vi "Main Loop.vi"(8 "error in (no error)":errorcluster, 11 "Sensor910 in":refnum<class "Sensor910.lvclass">) -> (0 "error out":errorcluster, 3 "Sensor910 out":refnum<class "Sensor910.lvclass">)   [LabVIEW 2020, in "Sensor910.lvclass"]
uses:
  Sensor910.lvclass
  <vilib>/Platform/TimedLoop/XDataNode/timing_clust.ctl
  <vilib>/Platform/TimedLoop/XDataNode/nitl_modes.ctl
  <vilib>/Platform/TimedLoop/XDataNode/wakeup.ctl
  Mode.ctl
  Command.ctl
  Settings.ctl
  Data.ctl
  9cfac15d-a9dc-4770-b8f0-68bacdc79c0f.vi
  94e3c92e-fcfa-43cb-ae47-d3a486abf537.vi
  b96c5f6a-59cc-4a84-9d2d-c86ca5fc82ce.vi
  9a13b59e-eb46-41c8-aff0-b09d3ab633f4.vi
  <vilib>/Platform/TimedLoop/scheduler/LVUserAPI/_suppVIs/Create_1kHz_TSource.vi
  <vilib>/NI Modbus.llb/MB Serial Master Query Write Single Register (poly).vi
  <vilib>/NI Modbus.llb/MB Serial Master Query Read Holding Registers (poly).vi
  <vilib>/NI Modbus.llb/MB Serial Master Query Read Input Registers (poly).vi
  <vilib>/platform/TimedLoop/XDataNode/XDataNode.xnode
  <vilib>/ErrorRing/Error Ring.xnode
  <vilib>/Platform/TimedLoop/XDataNode/XDNodeRunTimeDep.lvlib
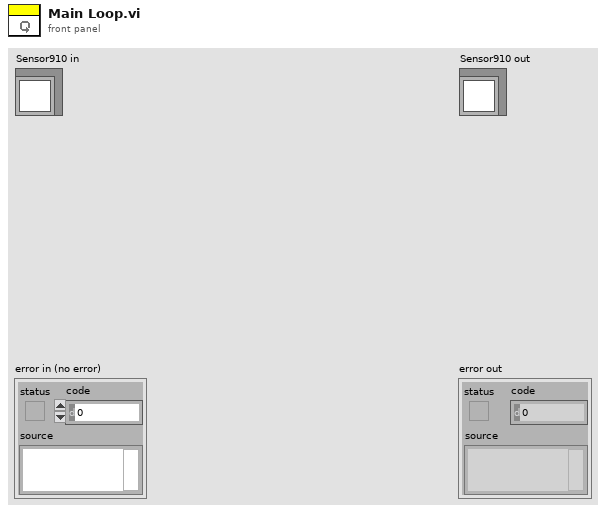
[diagram p1: front panel]
types:
  T1 = cluster{"Serial Parameters":cluster{"Mode":enum16{"RTU", "ASCII"}, "Slave Address":u8}, "VISA resource name":refnum<visa-resource-name>, "Period":i64, "Data Registers":u16[]}
  T2 = typedef "Sensor910.lvclass/Command.ctl" = cluster{"Address":u16, "Data":u16}
  T3 = typedef "Sensor910.lvclass/Settings.ctl" = cluster{"Serial Parameters":cluster{"Mode":enum16{"RTU", "ASCII"}, "Slave Address":u8}, "VISA resource name":refnum<visa-resource-name>, "Period":i64, "Data Registers":u16[], "Baud Rate":u32}
  T4 = typedef "Sensor910.lvclass/Data.ctl" = cluster{"Connect":bool, "No Response":bool, "Data":sgl[]}
  T5 = cluster{"Mode":enum16{"RTU", "ASCII"}, "Slave Address":u8}
  T6 = typedef "Sensor910.lvclass/Mode.ctl" = enum16{"Inactiv", "Read Data", "Service Mode", "Enter offset", "Open session", "Close session", "Set Modbus Address", "Abort"}
  T7 = typedef "XDNodeRunTimeDep.lvlib/timing_clust.ctl" = cluster{"Expected End [f-1]":u64, "Actual End [f-1]":u64, "Finished Late? [f-1]":bool, "Expected End [i-1]":u64, "Actual End [i-1]":u64, "Finished Late? [i-1]":bool, "Expected Start [i]":u64, "Actual Start [i]":u64, "Expected Start [f]":u64, "Actual Start [f]":u64, "Source Name":string, "Structure Name":string, "Period":i64, "Deadline":i64, "Offset":i64, "Start":i64, "Priority":i32, "Timeout":i32, "Mode":T8, "Wakeup Reason":T9, "Error":errorcluster, "Source Type":string, "Secondary Source Type":string, "Global End Time":u64, "Global Start Time":u64, "Frame Duration":u64, "Iteration Duration":u64, "Assigned CPU":i32, "I/O Scan Engine Mode":u32}
  T8 = typedef "XDNodeRunTimeDep.lvlib/nitl_modes.ctl" = enum32{"No Change", "Process missed periods, maintain original phase", "Discard missed periods, maintain original phase", "Process missed periods, ignore original phase", "Discard missed periods, ignore original phase"}
  T9 = typedef "XDNodeRunTimeDep.lvlib/wakeup.ctl" = enum32{"Normal", "Aborted", "Asynchronous wakeup", "Timing source error", "Timed loop error", "Timeout"}
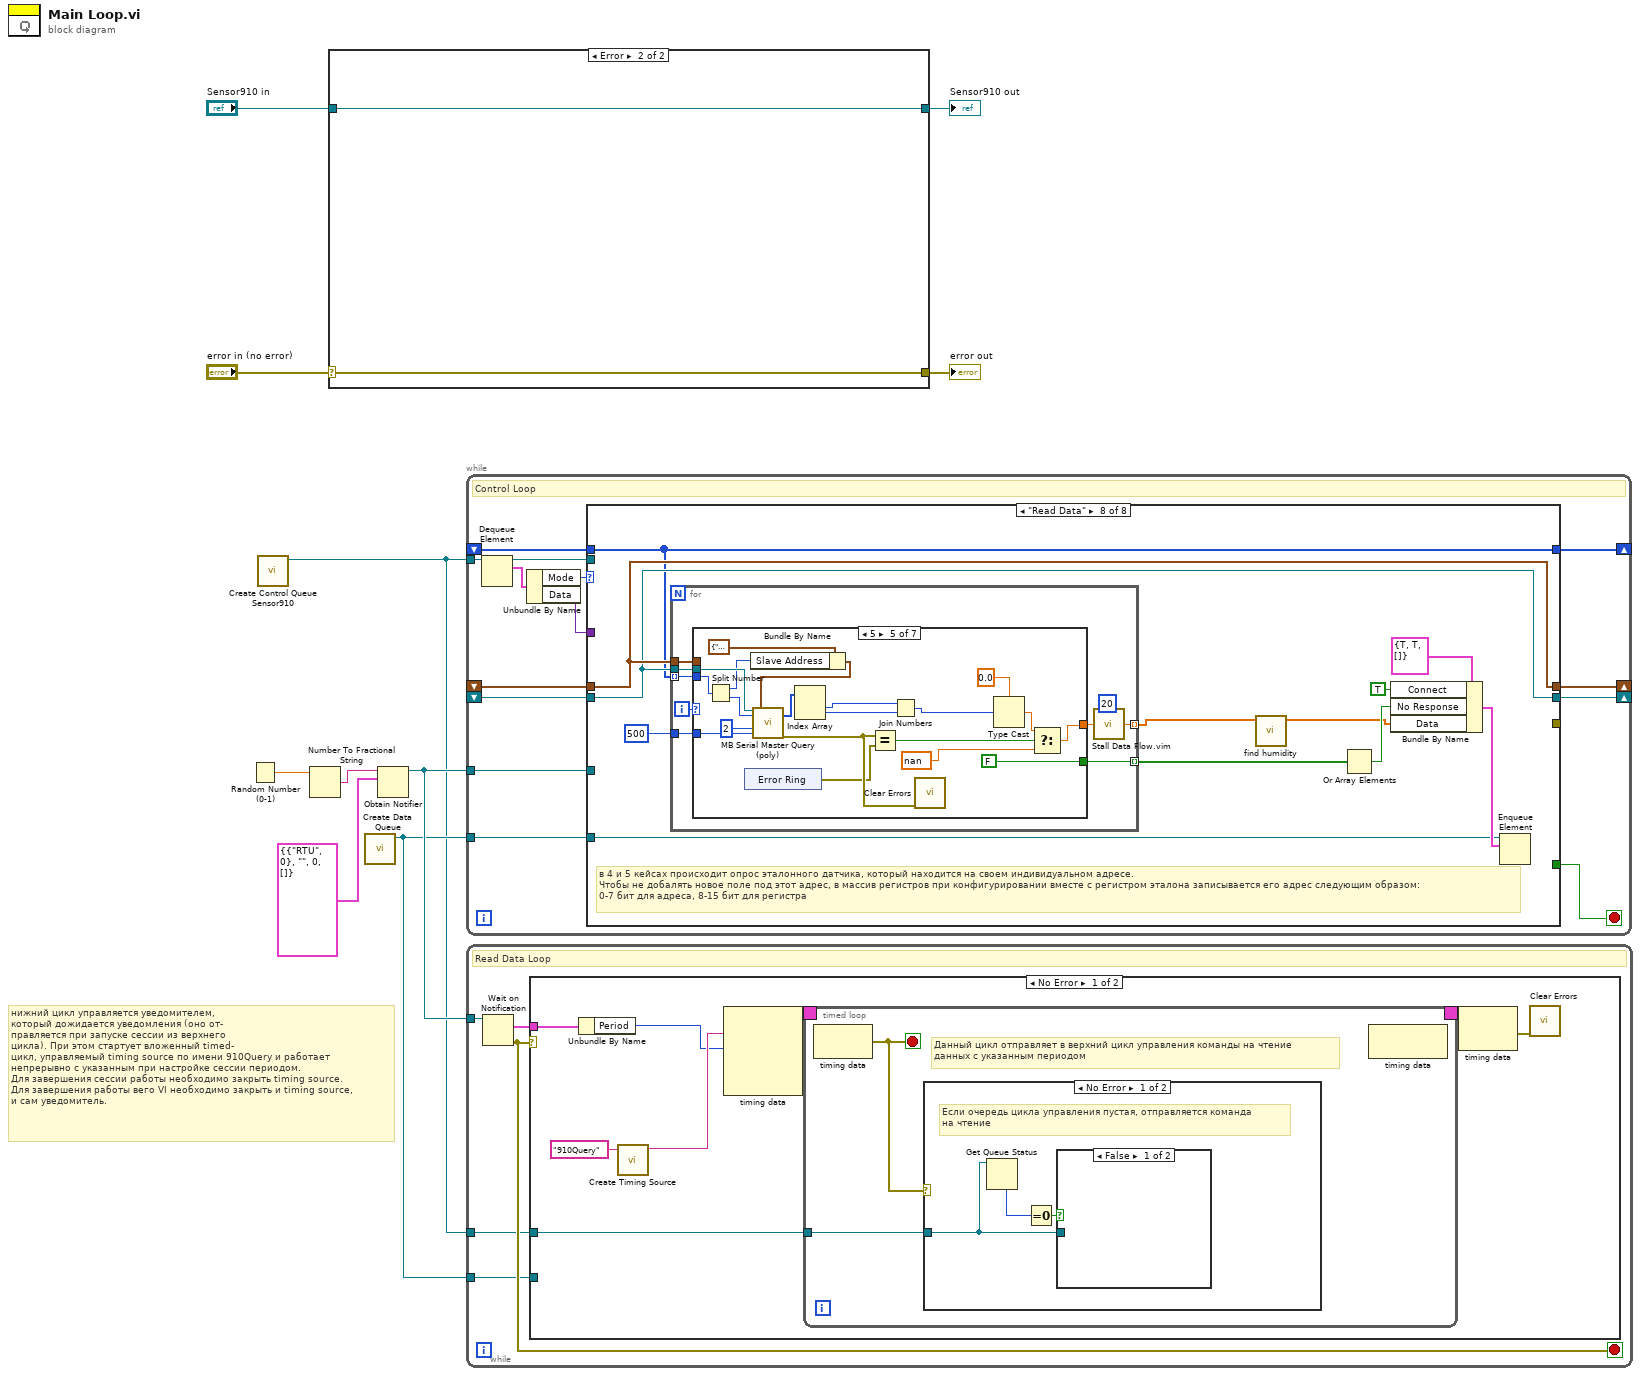
[diagram p0: block diagram]
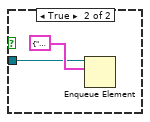
[diagram p2: hidden frame]
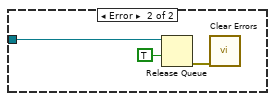
[diagram p4: hidden frame]
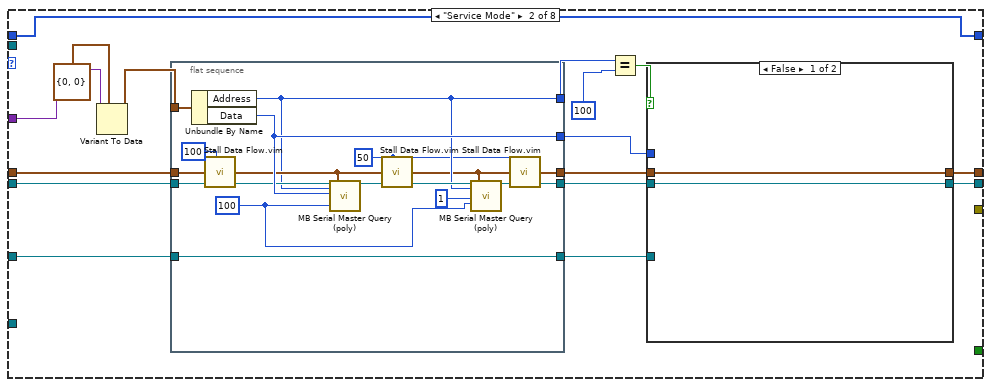
[diagram p6: hidden frame]
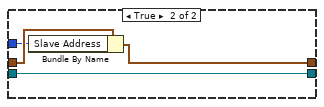
[diagram p7: hidden frame]
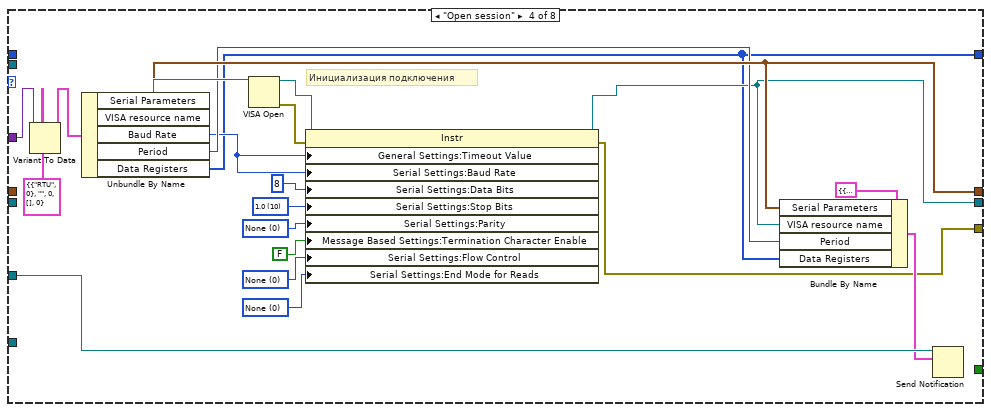
[diagram p9: hidden frame]
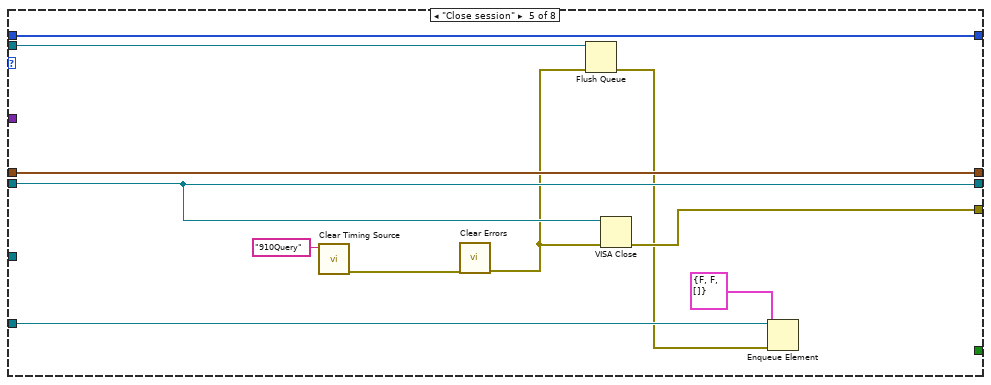
[diagram p10: hidden frame]
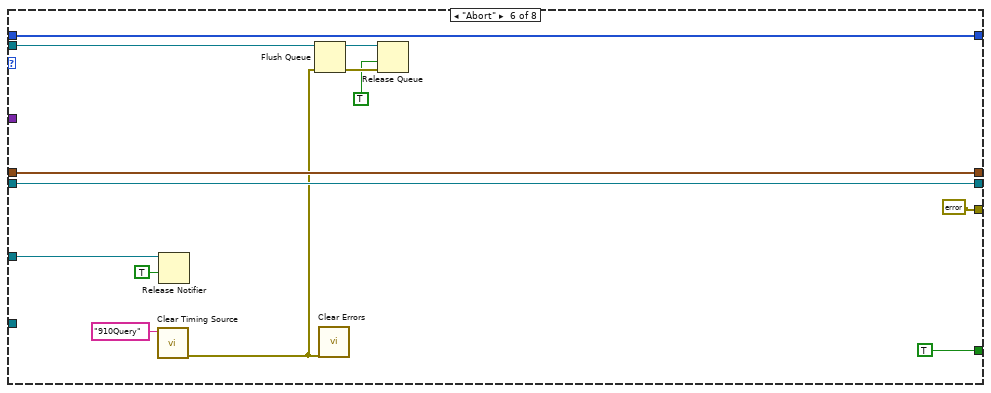
[diagram p11: hidden frame]
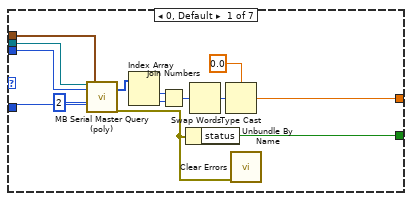
[diagram p13: hidden frame]
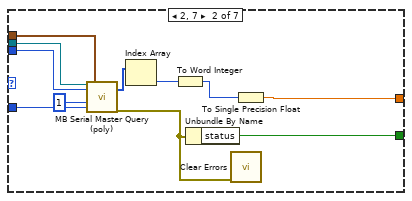
[diagram p14: hidden frame]
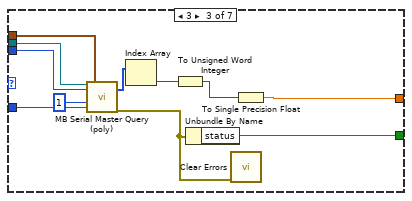
[diagram p15: hidden frame]
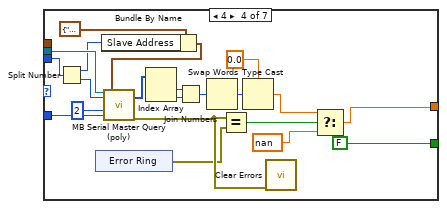
[diagram p16: hidden frame]
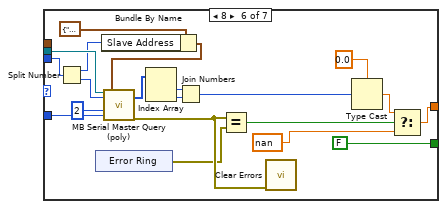
[diagram p17: hidden frame]
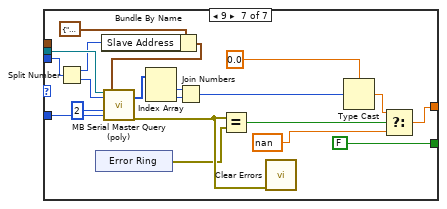
[diagram p18: hidden frame]
diagram:
  # "нижний цикл управляется уведомителем,\nкоторый дожидается уведомления (оно от-\nправляется при запуске сессии из верхнего\nцикла). При этом стартует вложенный timed-\nцикл, управляемый timing source по имени 910Query и работает\nнепрерывно с указанным при настройке сессии периодом.\nДля завершения сессии работы необходимо закрыть timing source.\nДля завершения работы вего VI необходимо закрыть и timing source,\nи сам уведомитель."
  n1 = Random Number (0-1)() -> (number: 0 to 1=w5:dbl)
  n2 = call "Create Control Queue Sensor910.vi"() -> ("queue out"=w1:refnum<queue>)  [unwired: 9 in, 2 out]
  n3 = Number To Fractional String(number=w5) -> (F-format string=w6:string)  [unwired: 3 in]
  n4 = case shown="Error" "error in (no error)" {
    selector: "error in (no error)" -> [w11 w14]
    tunnel: [w11 w14] -> w9
    tunnel: [w12 w13] -> w7
    tunnel: "Sensor910 in" -> [w12 w13]
    frame No Error {
      # "Wire the error cluster across even in the \"No Error\"\ncase so that warnings get propagated."
    }
    frame Error {
    }
  }
  "error out" <- w9
  "Sensor910 out" <- w7
  n5 = call "Create Data Queue.vi"() -> ("queue out"=w2:refnum<queue>)  [unwired: 10 in, 1 out]
  n6 = Obtain Notifier(name (unnamed)=w6, notification data type=T1 {"Serial Parameters"={"Mode"=enum."RTU", "Slave Address"=0}, "VISA resource name"="", "Period"=0, "Data Registers"=[]} ("Cluster")) -> (notifier out=w4:refnum<notifier>)  [unwired: 2 in, 2 out]
  n7 = while {
    tunnel: w1 -> [w28]
    tunnel: w4 -> [w25]
    shift-right: [w24] -> _
    shift-left: _ -> [w21]
    shift-right: [w23] -> _
    shift-left: _ -> [w20]
    shift-right: [w18] -> _
    shift-left: _ -> [w17]
    tunnel: w2 -> [w16]
    stop <- w19 stop-if-true
    # "Control Loop"
    n8 = Dequeue Element(queue=w28) -> (queue out=w15:refnum<queue>, element=w27:cluster{"Mode":T6, "Data":variant})  [unwired: 2 in, 2 out]
    n9 = Unbundle By Name(w27) -> ("Mode"=w26:T6, "Data"=w22:variant)
    n10 = case shown="\"Read Data\"" w26 {
      tunnel: w25 -> [_ w34 _ w83 _ w115 _ _]
      tunnel: [w31 w39 w71 w81 w101 w112 w118 w125] -> w24
      tunnel: [w30 w37 w70 w74 w100 w111 w119 w124] -> w23
      tunnel: w22 -> [_ w47 _ w79 _ _ _ _]
      tunnel: w21 -> [w31 w44 w71 _ w101 w112 w118 w125]
      tunnel: w20 -> [w30 w45 w70 _ w100 w111 w119 w124]
      tunnel: [_ _ _ w73 w99 errorcluster {"status"=TRUE, "code"=0, "source"=""} ("error out") _ _] -> _
      tunnel: [_ _ _ _ _ TRUE _ _] -> w19
      tunnel: [w29 w32 w69 w72 w98 w109 w117 w123] -> w18
      tunnel: w17 -> [w29 w32 w69 _ w98 w109 w117 w123]
      tunnel: w16 -> [_ _ _ _ w96 _ _ w122]
      tunnel: w15 -> [_ _ _ _ w95 w108 _ _]
      frame "Inactiv", Default {
      }
      frame "Service Mode" {
        n11 = Variant To Data(type=T2 {"Address"=0, "Data"=0} ("Command"), Variant=w47) -> (data=w43:T2)  [unwired: 1 in, 1 out]
        n12 = flat-sequence {
          tunnel: w45 -> [w63]
          tunnel: w44 -> [w65]
          tunnel: [w58] -> w36
          tunnel: w43 -> [w68]
          tunnel: [w56] -> w38
          tunnel: [w60] -> w42
          tunnel: [w67] -> w35
          tunnel: [w66] -> w33
          tunnel: w34 -> [w66]
          frame #0 {
            w55 = u32 50 ("milliseconds to wait")
            w54 = u32 100 ("Timeout")
            n13 = Unbundle By Name(w68) -> ("Address"=w60:u16, "Data"=w67:u16)
            n14 = call "Stall Data Flow.vim"("value in"=w65, "milliseconds to wait"=u32 100) -> ("value out"=w64:T5)  [unwired: 1 out]
            n15 = call-poly <vilib>:"MB Serial Master Query (poly).vi"("VISA resource name"=w63, "Address"=w60, "Holding Register"=w67, "Timeout"=w54, "Serial Parameters"=w64) -> ("VISA resource name out"=w61:refnum<visa-resource-name>)  [unwired: 12 in, 2 out]
            n16 = call "Stall Data Flow.vim"("value in"=w64, "milliseconds to wait"=w55) -> ("value out"=w57:T5)  [unwired: 1 out]
            n17 = call-poly <vilib>:"MB Serial Master Query (poly).vi"("VISA resource name"=w61, "Starting Address"=w60, "Quantity"=u16 1, "Timeout"=w54, "Serial Parameters"=w57) -> ("VISA resource name out"=w58:refnum<visa-resource-name>)  [unwired: 11 in, 3 out]
            n18 = call "Stall Data Flow.vim"("value in"=w57, "milliseconds to wait"=w55) -> ("value out"=w56:T5)  [unwired: 1 out]
          }
        }
        n19 = Equal?(x=w42, y=u16 100) -> (x = y?=w40:bool)
        n20 = case shown="False" w40 {
          tunnel: [w49 w50] -> w39
          tunnel: w38 -> [w49 w52]
          tunnel: [w48 w53] -> w37
          tunnel: w36 -> [w48 w53]
          tunnel: w35 -> [_ w51]
          tunnel: w33 -> [_ _]
          frame False {
          }
          frame True {
            n21 = Bundle By Name(cluster=w52, "Slave Address"=w51) -> (w50:T5)
          }
        }
      }
      frame "Enter offset" {
      }
      frame "Open session" {
        w92 = u16 0 items=["None", "Odd", "Even", "Mark", "Space"] ("Serial Settings:Parity")
        w91 = u16 0 items=["None", "XON/XOFF", "RTS/CTS", "XON/XOFF & RTS/CTS", "DTR/DSR", "XON/XOFF & DTR/DSR"] ("Serial Settings:Flow Control")
        w89 = u16 0 items=["None", "LastBit", "TermChar"] ("Serial Settings:Serial End Mode for Reads")
        w87 = u16 10 items=["1.0"=10, "1.5"=15, "2.0"=20] ("Serial Settings:Serial Stop Bits")
        # "Инициализация подключения"
        n22 = Variant To Data(type=T3 {"Serial Parameters"={"Mode"=enum."RTU", "Slave Address"=0}, "VISA resource name"="", "Period"=0, "Data Registers"=[], "Baud Rate"=0} ("Cluster"), Variant=w79) -> (data=w76:T3)  [unwired: 1 in, 1 out]
        n23 = Unbundle By Name(w76) -> ("Serial Parameters"=w81:T5, "VISA resource name"=w84:refnum<visa-resource-name>, "Baud Rate"=w77:u32, "Period"=w80:i64, "Data Registers"=w72:u16[])
        n24 = VISA Open(VISA resource name=w84) -> (VISA resource name=w86:refnum<visa-resource-name>, error out=w85:errorcluster)  [unwired: 4 in]
        n25 = property class="Instr"(reference=w86, error in=w85, "General Settings:Timeout Value"=w77, "Serial Settings:Baud Rate"=w77, "Serial Settings:Data Bits"=u16 8 ("data bits"), "Serial Settings:Stop Bits"=w87, "Serial Settings:Parity"=w92, "Message Based Settings:Termination Character Enable"=FALSE, "Serial Settings:Flow Control"=w91, "Serial Settings:End Mode for Reads"=w89) -> (reference out=w74:refnum<visa-resource-name>, error out=w73:errorcluster)
        n26 = Bundle By Name(cluster=T1 {"Serial Parameters"={"Mode"=enum."RTU", "Slave Address"=0}, "VISA resource name"="", "Period"=0, "Data Registers"=[]} ("notification"), "Serial Parameters"=w81, "VISA resource name"=w74, "Period"=w80, "Data Registers"=w72) -> (w75:T1)
        n27 = Send Notification(notification=w75, notifier=w83) -> ()  [unwired: 1 in, 2 out]
      }
      frame "Close session" {
        n28 = call <vilib>:"Clear Timing Source.vi"("name"="910Query" ("name (in)")) -> ("error out"=w102:errorcluster)  [unwired: 9 in, 1 out]
        n29 = call <vilib>:"Clear Errors.vi"("error in (no error)"=w102) -> ("error out"=w94:errorcluster)  [unwired: 5 in, 1 out]
        n30 = Flush Queue(queue=w95, error in (no error)=w94) -> (error out=w93:errorcluster)  [unwired: 2 out]
        n31 = VISA Close(VISA resource name=w100, error in (no error)=w94) -> (error out=w99:errorcluster)
        n32 = Enqueue Element(queue=w96, element=T4 {"Connect"=FALSE, "No Response"=FALSE, "Data"=[]}, error in (no error)=w93) -> ()  [unwired: 1 in, 3 out]
      }
      frame "Abort" {
        n33 = call <vilib>:"Clear Timing Source.vi"("name"="910Query" ("name (in)")) -> ("error out"=w107:errorcluster)  [unwired: 9 in, 1 out]
        n34 = Release Notifier(notifier=w115, force destroy? (F)=TRUE) -> ()  [unwired: 1 in, 3 out]
        n35 = Flush Queue(queue=w108, error in (no error)=w107) -> (queue out=w106:refnum<queue>, error out=w105:errorcluster)  [unwired: 1 out]
        n36 = call <vilib>:"Clear Errors.vi"("error in (no error)"=w107) -> ()  [unwired: 5 in, 2 out]
        n37 = Release Queue(queue=w106, force destroy? (F)=TRUE, error in (no error)=w105) -> ()  [unwired: 3 out]
      }
      frame "Set Modbus Address" {
      }
      frame "Read Data" {
        # "в 4 и 5 кейсах происходит опрос эталонного датчика, который находится на своем индивидуальном адресе.\nЧтобы не добалять новое поле под этот адрес, в массив регистров при конфигурировании вместе с регистром эталона записывается его адрес следующим образом:\n0-7 бит для адреса, 8-15 бит для регистра"
        n38 = for {
          tunnel: w125 -> [w140]
          tunnel: w124 -> [w139]
          tunnel: w123 -> [w138] mode=indexing
          tunnel: [w134] -> w130 mode=indexing
          tunnel: [w137] -> w128 mode=indexing
          tunnel: u32 500 ("Timeout") -> [w132]
          i -> [w136]
          n39 = case shown="5" w136 {
            tunnel: w140 -> [w154 w165 w176 _ _ _ _]
            tunnel: w139 -> [w153 w164 w175 w197 w218 w239 w260]
            tunnel: w138 -> [w152 w163 w174 w194 w215 w236 w257]
            tunnel: [w145 w158 w170 w179 w206 w224 w245] -> w135
            tunnel: [w143 w161 w173 FALSE ("status") FALSE ("status") FALSE ("status") FALSE ("status")] -> w137
            tunnel: w132 -> [w141 w155 w166 w177 w204 w222 w243]
            frame 0, Default {
              n40 = call-poly <vilib>:"MB Serial Master Query (poly).vi"("VISA resource name"=w153, "Starting Address"=w152, "Quantity"=u16 2, "Timeout"=w141, "Serial Parameters"=w154) -> ("Holding Registers"=w146:u16[], "error out"=w144:errorcluster)  [unwired: 11 in, 2 out]
              n41 = Index Array(array=w146) -> (element #1=w149:u16, element #2=w147:u16)  [unwired: 2 in]
              n42 = Join Numbers(hi=w149, lo=w147) -> ((hi.lo)=w151:u32)
              n43 = Unbundle By Name(w144) -> ("status"=w143:bool)
              n44 = Swap Words(1:w151) -> (0:w150:u32)
              n45 = Type Cast(type=sgl 0.0 ("p_atm"), x=w150) -> (*(type *) &x=w145:sgl)
              n46 = call <vilib>:"Clear Errors.vi"("error in (no error)"=w144) -> ()  [unwired: 5 in, 2 out]
            }
            frame 2, 7 {
              n47 = call-poly <vilib>:"MB Serial Master Query (poly).vi"("VISA resource name"=w164, "Starting Address"=w163, "Quantity"=u16 1, "Timeout"=w155, "Serial Parameters"=w165) -> ("Holding Registers"=w159:u16[], "error out"=w162:errorcluster)  [unwired: 11 in, 2 out]
              n48 = Index Array(array=w159) -> (element=w157:u16)  [unwired: 1 in]
              n49 = To Word Integer(number=w157) -> (16bit integer=w156:i16)
              n50 = Unbundle By Name(w162) -> ("status"=w161:bool)
              n51 = call <vilib>:"Clear Errors.vi"("error in (no error)"=w162) -> ()  [unwired: 5 in, 2 out]
              n52 = To Single Precision Float(number=w156) -> (single precision float=w158:sgl)
            }
            frame 3 {
              n53 = call-poly <vilib>:"MB Serial Master Query (poly).vi"("VISA resource name"=w175, "Starting Address"=w174, "Quantity"=u16 1, "Timeout"=w166, "Serial Parameters"=w176) -> ("Holding Registers"=w171:u16[], "error out"=w167:errorcluster)  [unwired: 11 in, 2 out]
              n54 = Index Array(array=w171) -> (element=w169:u16)  [unwired: 1 in]
              n55 = To Unsigned Word Integer(number=w169) -> (unsigned 16bit integer=w168:u16)
              n56 = Unbundle By Name(w167) -> ("status"=w173:bool)
              n57 = call <vilib>:"Clear Errors.vi"("error in (no error)"=w167) -> ()  [unwired: 5 in, 2 out]
              n58 = To Single Precision Float(number=w168) -> (single precision float=w170:sgl)
            }
            frame 4 {
              n59 = Split Number(x=w194) -> (hi(x)=w193:u8, lo(x)=w192:u8)
              n60 = xnode "Error Ring"() -> ("error out"=w182:errorcluster)
              n61 = Bundle By Name(cluster=T5 {"Mode"=enum."RTU", "Slave Address"=0} ("Serial Parameters"), "Slave Address"=w193) -> (w191:T5)
              n62 = call-poly <vilib>:"MB Serial Master Query (poly).vi"("VISA resource name"=w197, "Starting Address"=w192, "Quantity"=u16 2, "Timeout"=w177, "Serial Parameters"=w191) -> ("Input Registers"=w185:u16[], "error out"=w183:errorcluster)  [unwired: 11 in, 2 out]
              n63 = Index Array(array=w185) -> (element #1=w188:u16, element #2=w186:u16)  [unwired: 2 in]
              n64 = Join Numbers(hi=w188, lo=w186) -> ((hi.lo)=w190:u32)
              n65 = Swap Words(1:w190) -> (0:w189:u32)
              n66 = Equal?(x=w183, y=w182) -> (x = y?=w180:bool)
              n67 = Type Cast(type=sgl 0.0 ("p_atm"), x=w189) -> (*(type *) &x=w181:sgl)
              n68 = call <vilib>:"Clear Errors.vi"("error in (no error)"=w183) -> ()  [unwired: 5 in, 2 out]
              n69 = Select(t=w181, s=w180, f=sgl nan) -> (s? t:f=w179:sgl)
            }
            frame 5 {
              n70 = Split Number(x=w215) -> (hi(x)=w214:u8, lo(x)=w213:u8)
              n71 = xnode "Error Ring"() -> ("error out"=w208:errorcluster)
              n72 = Bundle By Name(cluster=T5 {"Mode"=enum."RTU", "Slave Address"=0} ("Serial Parameters"), "Slave Address"=w214) -> (w212:T5)
              n73 = call-poly <vilib>:"MB Serial Master Query (poly).vi"("VISA resource name"=w218, "Starting Address"=w213, "Quantity"=u16 2, "Timeout"=w204, "Serial Parameters"=w212) -> ("Holding Registers"=w210:u16[], "error out"=w209:errorcluster)  [unwired: 11 in, 2 out]
              n74 = Index Array(array=w210) -> (element #1=w200:u16, element #2=w199:u16)  [unwired: 2 in]
              n75 = Equal?(x=w209, y=w208) -> (x = y?=w207:bool)
              n76 = Join Numbers(hi=w200, lo=w199) -> ((hi.lo)=w201:u32)
              n77 = call <vilib>:"Clear Errors.vi"("error in (no error)"=w209) -> ()  [unwired: 5 in, 2 out]
              n78 = Type Cast(type=sgl 0.0 ("p_atm"), x=w201) -> (*(type *) &x=w202:sgl)
              n79 = Select(t=w202, s=w207, f=sgl nan) -> (s? t:f=w206:sgl)
            }
            frame 8 {
              n80 = Split Number(x=w236) -> (hi(x)=w235:u8, lo(x)=w234:u8)
              n81 = xnode "Error Ring"() -> ("error out"=w227:errorcluster)
              n82 = Bundle By Name(cluster=T5 {"Mode"=enum."RTU", "Slave Address"=0} ("Serial Parameters"), "Slave Address"=w235) -> (w233:T5)
              n83 = call-poly <vilib>:"MB Serial Master Query (poly).vi"("VISA resource name"=w239, "Starting Address"=w234, "Quantity"=u16 2, "Timeout"=w222, "Serial Parameters"=w233) -> ("Holding Registers"=w229:u16[], "error out"=w228:errorcluster)  [unwired: 11 in, 2 out]
              n84 = Index Array(array=w229) -> (element #1=w232:u16, element #2=w230:u16)  [unwired: 2 in]
              n85 = Join Numbers(hi=w232, lo=w230) -> ((hi.lo)=w220:u32)
              n86 = Equal?(x=w228, y=w227) -> (x = y?=w225:bool)
              n87 = call <vilib>:"Clear Errors.vi"("error in (no error)"=w228) -> ()  [unwired: 5 in, 2 out]
              n88 = Type Cast(type=sgl 0.0 ("p_atm"), x=w220) -> (*(type *) &x=w226:sgl)
              n89 = Select(t=w226, s=w225, f=sgl nan) -> (s? t:f=w224:sgl)
            }
            frame 9 {
              n90 = Split Number(x=w257) -> (hi(x)=w256:u8, lo(x)=w255:u8)
              n91 = xnode "Error Ring"() -> ("error out"=w248:errorcluster)
              n92 = Bundle By Name(cluster=T5 {"Mode"=enum."RTU", "Slave Address"=0} ("Serial Parameters"), "Slave Address"=w256) -> (w254:T5)
              n93 = call-poly <vilib>:"MB Serial Master Query (poly).vi"("VISA resource name"=w260, "Starting Address"=w255, "Quantity"=u16 2, "Timeout"=w243, "Serial Parameters"=w254) -> ("Holding Registers"=w250:u16[], "error out"=w249:errorcluster)  [unwired: 11 in, 2 out]
              n94 = Index Array(array=w250) -> (element #1=w253:u16, element #2=w251:u16)  [unwired: 2 in]
              n95 = Join Numbers(hi=w253, lo=w251) -> ((hi.lo)=w241:u32)
              n96 = Equal?(x=w249, y=w248) -> (x = y?=w246:bool)
              n97 = call <vilib>:"Clear Errors.vi"("error in (no error)"=w249) -> ()  [unwired: 5 in, 2 out]
              n98 = Type Cast(type=sgl 0.0 ("p_atm"), x=w241) -> (*(type *) &x=w247:sgl)
              n99 = Select(t=w247, s=w246, f=sgl nan) -> (s? t:f=w245:sgl)
            }
          }
          n100 = call "Stall Data Flow.vim"("value in"=w135, "milliseconds to wait"=u32 20) -> ("value out"=w134:sgl)  [unwired: 1 out]
        }
        n101 = call "find humidity.vi"("Array in"=w130) -> ("Array out"=w120:sgl[])  [unwired: 10 in]
        n102 = Or Array Elements(Boolean array=w128) -> (logical OR=w129:bool)
        n103 = Bundle By Name(cluster=T4 {"Connect"=TRUE, "No Response"=TRUE, "Data"=[]} ("Data"), "Connect"=TRUE, "No Response"=w129, "Data"=w120) -> (w131:T4)
        n104 = Enqueue Element(queue=w122, element=w131) -> ()  [unwired: 2 in, 3 out]
      }
    }
  }
  n105 = while {
    tunnel: w4 -> [w266]
    tunnel: w2 -> [w263]
    tunnel: w1 -> [w262]
    stop <- w264 stop-if-true
    # "Read Data Loop"
    n106 = Wait on Notification(notifier=w266) -> (notification=w265:T1, error out=w264:errorcluster)  [unwired: 3 in, 2 out]
    n107 = case shown="No Error" w264 {
      tunnel: w265 -> [w272 _]
      tunnel: w263 -> [_ w291]
      tunnel: w262 -> [w267 _]
      frame No Error {
        n108 = Unbundle By Name(w272) -> ("Period"=w269:i64)
        n109 = call-poly <vilib>:"Create Timing Source.vi"("name (in)"="910Query") -> ("name (out)"=w270:string)  [unwired: 9 in, 1 out]
        n110 = node-c288(w270, w269) -> (w274:T7)  [unwired: 2 in]
        n111 = timed-loop {
          timing: w274 -> [_]
          timing-out: [_] -> w273
          tunnel: w267 -> [w276]
          stop <- w275 stop-if-true
          # "Данный цикл отправляет в верхний цикл управления команды на чтение\nданных с указанным периодом"
          n112 = node-c288() -> (w275:errorcluster)  [unwired: 1 in]
          n113 = case shown="No Error" w275 {
            tunnel: w276 -> [w279 _]
            frame No Error {
              # "Если очередь цикла управления пустая, отправляется команда\nна чтение"
              n114 = Get Queue Status(queue=w279) -> (# elements in queue=w278:i32)  [unwired: 2 in, 7 out]
              n115 = Equal To 0?(x=w278) -> (x = 0?=w277:bool)
              n116 = case shown="False" w277 {
                tunnel: w279 -> [_ w280]
                frame False {
                }
                frame True {
                  n117 = Enqueue Element(queue=w280, element=cluster{"Mode":T6, "Data":variant} {"Mode"=enum."Read Data", "Data"=variant}) -> ()  [unwired: 2 in, 3 out]
                }
              }
            }
            frame Error {
            }
          }
          n118 = node-c288() -> ()  [unwired: 1 in, 1 out]
        }
        n119 = node-c288(w273) -> (w268:errorcluster)
        n120 = call <vilib>:"Clear Errors.vi"("error in (no error)"=w268) -> ()  [unwired: 5 in, 2 out]
      }
      frame Error {
        n121 = Release Queue(queue=w291, force destroy? (F)=TRUE) -> (error out=w292:errorcluster)  [unwired: 1 in, 2 out]
        n122 = call <vilib>:"Clear Errors.vi"("error in (no error)"=w292) -> ()  [unwired: 5 in, 2 out]
      }
    }
  }
